vi "DetermineCompositionInput.vi"(8 "error in (no error)":errorcluster, 11 "SMO.UI.MAUI in":refnum<class "MAUI.lvclass">) -> (0 "error out":errorcluster, 1 "Is Path?":bool, 2 "Composition Input":string, 3 "SMO.UI.MAUI out":refnum<class "MAUI.lvclass">, 4 "Valid Input?":bool)   [LabVIEW 2019, in "MAUI.lvclass"]
doc: "If it is composition, then it will determine if the application name or path was provided. If it is neither of these, then it will be considered invalid input."
uses:
  MAUI.lvclass
  MAUI.lvclass/MAUI.ctl
  <vilib>/Utility/Data Type/NI_Data Type.lvlib
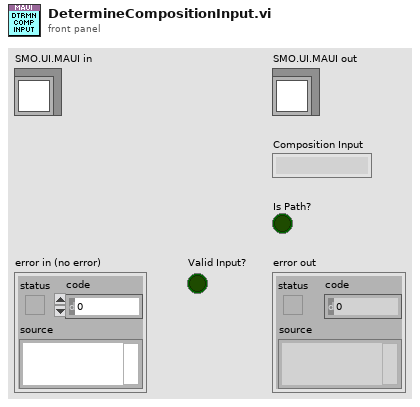
[diagram p1: front panel]
types:
  T1 = typedef "NI_Data Type.lvlib/Data Type.ctl" = enum8{"Invalid Type", "Void", "I8", "I16", "I32", "I64", "U8", "U16", "U32", "U64", "Single Float", "Double Float", "Extended Float", "Single Complex", "Double Complex", "Extended Complex", "Enum U8", "Enum U16", "Enum U32", "Enum U64", "Single Float With Unit", "Double Float With Unit", "Extended Float With Unit", "Single Complex with Unit", "Double Complex with Unit", "Extended Complex with Unit", "Boolean", "String", "Path", "Picture", "Tag", "Array", "Cluster", "Variant", "LV Variant", "Waveform", "Timestamp", "Digital Waveform", "Digital Data", "ExpressData", "Refnum", "External Data", "VI", "Poly VI", "LabVIEW Class Instance", "Fixed Point", "Set Collection", "Map Collection"}
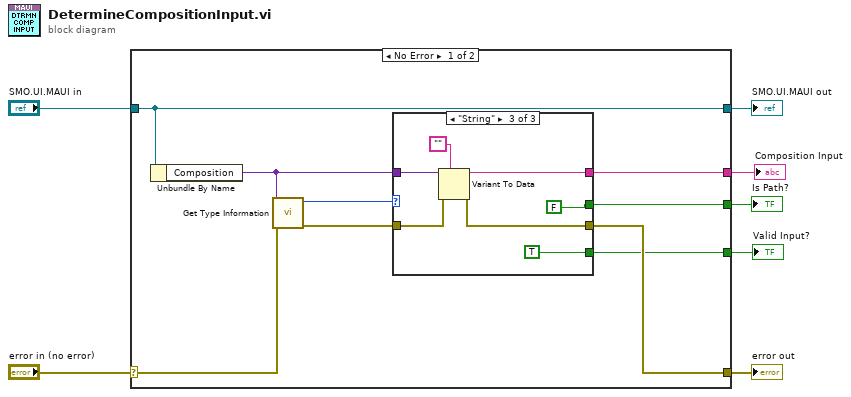
[diagram p0: block diagram]
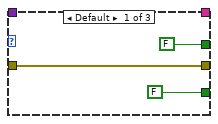
[diagram p2: hidden frame]
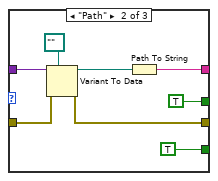
[diagram p3: hidden frame]
diagram:
  n1 = case shown="No Error" "error in (no error)" {
    selector: "error in (no error)" -> [w16 w36]
    tunnel: [w14 w36] -> w6
    tunnel: [w13 w35] -> w4
    tunnel: "SMO.UI.MAUI in" -> [w13 w35]
    tunnel: [w11 _] -> w3
    tunnel: [w9 _] -> w2
    tunnel: [w8 _] -> w1
    frame No Error {
      n2 = Unbundle By Name(w13) -> ("Composition"=w10:variant)
      n3 = call <vilib>:"Get Type Information.vi"("error in (no error)"=w16, "variant"=w10) -> ("error out"=w15:errorcluster, "type"=w12:T1)  [unwired: 5 in, 3 out]
      n4 = case shown="\"String\"" w12 {
        tunnel: [FALSE TRUE TRUE] -> w11
        tunnel: w10 -> [_ w24 w31]
        tunnel: [_ w21 w29] -> w9
        tunnel: w15 -> [w19 w27 w34]
        tunnel: [w19 w26 w33] -> w14
        tunnel: [FALSE TRUE FALSE] -> w8
        frame Default {
        }
        frame "Path" {
          n5 = Variant To Data(error in=w27, type=path "", Variant=w24) -> (data=w22:path, error out=w26:errorcluster)
          n6 = Path To String(path=w22) -> (string=w21:string)
        }
        frame "String" {
          n7 = Variant To Data(error in=w34, type="", Variant=w31) -> (data=w29:string, error out=w33:errorcluster)
        }
      }
    }
    frame Error {
    }
  }
  "error out" <- w6
  "SMO.UI.MAUI out" <- w4
  "Valid Input?" <- w3
  "Composition Input" <- w2
  "Is Path?" <- w1
